vi "ReadLockGlobals.vi"() -> ()   [LabVIEW 2019]
panel:
  out "Fresh":bool[](array[boolean])
  out "Array 2":dbl[](array[numeric])
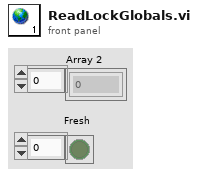
[diagram p1: front panel]
diagram:
